vi "Air Intake Dynamics.vi"(9 "dt":sgl=1.0 format="%0.2f", 10 "Engine Speed (rad/s)":sgl, 11 "Throttle Angle (deg)":sgl) -> (2 "Air Mass/Cycle (g)":sgl, 3 "Manifold Pressure (bar)":sgl format="%0.2f")   [LabVIEW 2016, in "NI-PCG Vehicle Model.lvlib"]
uses:
  NI-PCG Vehicle Model.lvlib
  Globals/Parameters.vi
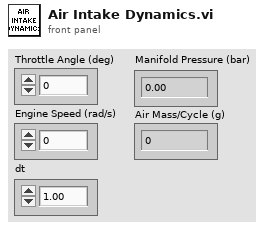
[diagram p1: front panel]
types:
  T1 = typedef "NI-PCG Vehicle Model.lvlib/Engine Parameters.ctl" = cluster{"Ambient Parameters":cluster{"Temperature (K)":sgl, "Pressure (Pa)":sgl}, "Air Parameters":cluster{"R (Ideal Gas Constant)":sgl, "Molecular Weight":sgl, "Cp (Specific Heat Constant)":sgl, "Density (kg/m^3)":sgl, "Stoichiometric A/F Ratio":sgl}, "Engine Geometry Parameters":cluster{"Cylinder Volume (l)":sgl, "J (Rotational Moment of Inertia)":sgl, "Minimuim Engine Speed":sgl, "Maximum Engine Speed":sgl, "Intake Manifold Volume (l)":sgl}, "Volumetric Efficiency Map":cluster{"MAP":sgl[], "RPM":sgl[], "Table":sgl[][]}, "Fuel LHV (J/kg)":sgl, "Combustion Efficiency Map":cluster{"Spark Timing (deg BTDC))":sgl[], "Engine Speed (RPM)":sgl[], "Combustion Efficiency":sgl[][]}, "Thermodynamic Efficiency":sgl}
  T2 = typedef "NI-PCG Vehicle Model.lvlib/Transmission Parameters.ctl" = cluster{"Final Drive Ratio":sgl, "Transmission Gear Ratios":cluster{"Gears":sgl[], "Gear Ratios":sgl[]}, "Torque Converter Map":cluster{"Speed Ratio":sgl[], "K Factor":sgl[], "Torque Ratio":sgl[]}, "Upshift Throttle":sgl[], "Downshift Throttle":sgl[], "Upshift Table":sgl[][], "Downshift Table":sgl[][], "Wait Time":u8}
  T3 = typedef "NI-PCG Vehicle Model.lvlib/Vehicle Parameters.ctl" = cluster{"Vehicle Mass (kg)":sgl, "Vehicle Cd":sgl, "Vehicle Frontal Area (m^2)":sgl, "Wheel Radius (m)":sgl, "Wheel Rolling Resistance":sgl}
  T4 = cluster{"Engine Parameters":T1, "Transmission Parameters":T2, "Vehicle Parameters":T3}
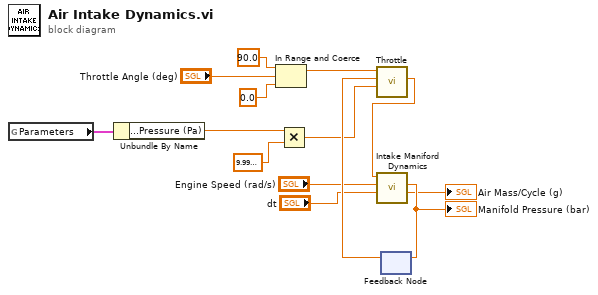
[diagram p0: block diagram]
diagram:
  n1 = global read "Parameters.vi" "Parameters"() -> (w1:T4)
  n2 = Unbundle By Name(w1) -> ("Engine Parameters.Ambient Parameters.Pressure (Pa)"=w8:sgl)
  n3 = In Range and Coerce(upper limit=sgl 90.0, x="Throttle Angle (deg)", lower limit=sgl 0.0) -> (coerced(x)=w14:sgl)  [unwired: 1 out]
  n4 = Multiply(x=w8, y=sgl 1e-05) -> (x*y=w6:sgl)
  n5 = feedback #1() -> (w9:sgl)  [unwired: 1 in]
  n6 = call "Throttle.vi"("Atmospheric Pressure (bar)"=w6, "Manifold Pressure (bar)"=w9, "Throttle Angle (deg)"=w14) -> ("Throttle Flow (g/s)"=w5:sgl)  [unwired: 8 in]
  n7 = call "Intake Maniford Dynamics.vi"("dt"="dt", "Engine Speed (rad/s)"="Engine Speed (rad/s)", "Air Mass Flow from Throttle (g/s)"=w5) -> ("Air Mass/Cycle (g)"=→"Air Mass/Cycle (g)":sgl, "Manifold Pressure (bar)"=w10:sgl)  [unwired: 6 in, 1 out]
  "Manifold Pressure (bar)" <- w10
  n8 = feedback-in #1(w10) -> ()
